vi "open with serial number.vi"(8 "error in (no error)":errorcluster caption="entrée d'erreur (pas d'erreur)", 10 "len":u32, 11 "serial_number":string) -> (0 "error out":errorcluster caption="sortie d'erreur", 3 "Handle":i32)   [LabVIEW 2020, in "usb_relay_device.lvlib"]
doc: "int EXPORT_API usb_relay_device_open_with_serial_number(const char *serial_number, unsigned len);"
uses:
  usb_relay_device.lvlib
  usb_relay_device.dll
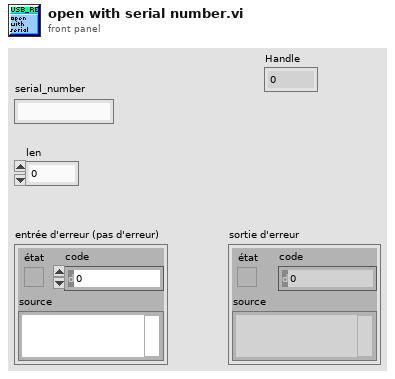
[diagram p1: front panel]
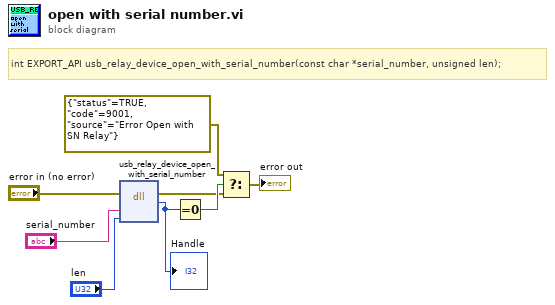
[diagram p0: block diagram]
diagram:
  # "int EXPORT_API usb_relay_device_open_with_serial_number(const char *serial_number, unsigned len);"
  n1 = dll-call lib="C:/Users/ngarcin/OneDrive - Altyor/Standard TB/Class/Relay_Board/Relay_Board usb_Relay_device/usb_relay_device/usb_relay_device.dll" fn="usb_relay_device_open_with_serial_number"(error in="error in (no error)", "serial_number"="serial_number", "len"="len") -> (error out=w2:errorcluster, "type de retour"=w3:i32)  [unwired: 4 in, 1 out]
  "Handle" <- w3
  n2 = Equal To 0?(x=w3) -> (x = 0?=w5:bool)
  n3 = Select(t=errorcluster {"status"=TRUE, "code"=9001, "source"="Error Open with SN Relay"} ("sortie d'erreur"), s=w5, f=w2) -> (s? t:f=→"error out":errorcluster)
